vi "Place Hatch Auto.vi"   [LabVIEW 2018]
uses:
  SubSystems/Hatch Panel Intake/Hatch Panel Intake Global.vi
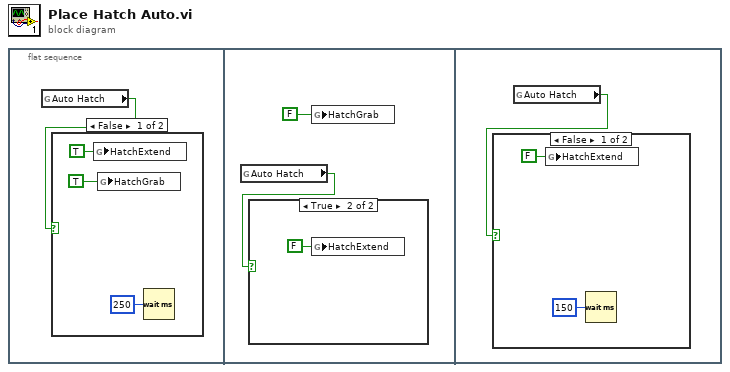
[diagram p0: block diagram]
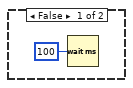
[diagram p3: hidden frame]
diagram:
  n1 = flat-sequence {
    frame #0 {
      n2 = global read "Hatch Panel Intake Global.vi" "Auto Hatch"() -> (w1:bool)
      n3 = case shown="False" w1 {
        frame False {
          n4 = global write "Hatch Panel Intake Global.vi" "HatchExtend"(TRUE ("HatchExtend")) -> ()
          n5 = global write "Hatch Panel Intake Global.vi" "HatchGrab"(TRUE ("HatchExtend")) -> ()
          n6 = Wait (ms)(milliseconds to wait=u32 250) -> ()  [unwired: 1 out]
        }
        frame True {
        }
      }
    }
    frame #1 {
      n7 = global read "Hatch Panel Intake Global.vi" "Auto Hatch"() -> (w5:bool)
      n8 = case shown="True" w5 {
        frame False {
          n9 = Wait (ms)(milliseconds to wait=u32 100) -> ()  [unwired: 1 out]
        }
        frame True {
          n10 = global write "Hatch Panel Intake Global.vi" "HatchExtend"(FALSE ("HatchExtend")) -> ()
        }
      }
      n11 = global write "Hatch Panel Intake Global.vi" "HatchGrab"(FALSE ("HatchExtend")) -> ()
    }
    frame #2 {
      n12 = global read "Hatch Panel Intake Global.vi" "Auto Hatch"() -> (w9:bool)
      n13 = case shown="False" w9 {
        frame False {
          n14 = global write "Hatch Panel Intake Global.vi" "HatchExtend"(FALSE ("HatchExtend")) -> ()
          n15 = Wait (ms)(milliseconds to wait=u32 150) -> ()  [unwired: 1 out]
        }
        frame True {
        }
      }
    }
  }
